vi "Send VmaxVmin Notifier.vi"(8 "error in (no error)":errorcluster, 9 "VmaxVmin Range":string, 10 "Channel":string) -> (0 "error out":errorcluster)   [LabVIEW 2015]
uses:
  DAQ Engine VIs/PXI Globals.vi
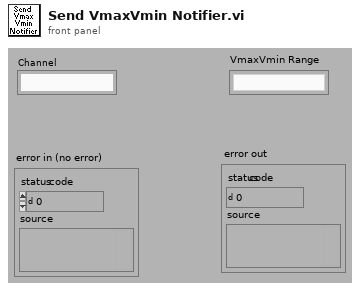
[diagram p1: front panel]
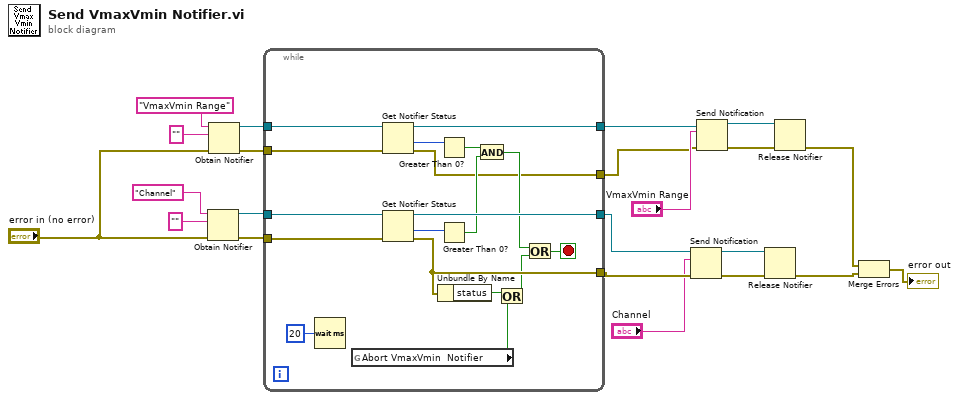
[diagram p0: block diagram]
diagram:
  n1 = Obtain Notifier(name (unnamed)="Channel", notification data type="" ("Channel 2"), error in (no error)="error in (no error)") -> (notifier out=w14:refnum<notifier>, error out=w13:errorcluster)  [unwired: 1 in, 1 out]
  n2 = Obtain Notifier(name (unnamed)="VmaxVmin Range", notification data type="" ("Channel 2"), error in (no error)="error in (no error)") -> (notifier out=w9:refnum<notifier>, error out=w10:errorcluster)  [unwired: 1 in, 1 out]
  n3 = while {
    tunnel: w14 -> [w39]
    tunnel: w13 -> [w38]
    tunnel: [w36] -> w15
    tunnel: [w26] -> w16
    tunnel: w10 -> [w33]
    tunnel: w9 -> [w32]
    tunnel: [w28] -> w5
    tunnel: [w27] -> w4
    stop <- w35 stop-if-true
    n4 = Wait (ms)(milliseconds to wait=20) -> ()  [unwired: 1 out]
    n5 = global read "PXI Globals.vi" "Abort VmaxVmin  Notifier"() -> (w24:bool)
    n6 = Get Notifier Status(notifier=w32, error in (no error)=w33) -> (notifier out=w28:refnum<notifier>, # waiting=w34:i32, error out=w27:errorcluster)  [unwired: 2 out]
    n7 = Get Notifier Status(notifier=w39, error in (no error)=w38) -> (notifier out=w36:refnum<notifier>, # waiting=w37:i32, error out=w26:errorcluster)  [unwired: 2 out]
    n8 = Unbundle By Name(w26) -> ("status"=w25:bool)
    n9 = Greater Than 0?(x=w34) -> (x > 0?=w31:bool)
    n10 = Greater Than 0?(x=w37) -> (x > 0?=w30:bool)
    n11 = And(x=w31, y=w30) -> (x .and. y?=w29:bool)
    n12 = Or(x=w25, y=w24) -> (x .or. y?=w23:bool)
    n13 = Or(x=w29, y=w23) -> (x .or. y?=w35:bool)
  }
  n14 = Send Notification(notification="Channel", notifier=w15, error in (no error)=w16) -> (notifier out=w17:refnum<notifier>, error out=w18:errorcluster)
  n15 = Send Notification(notification="VmaxVmin Range", notifier=w5, error in (no error)=w4) -> (notifier out=w7:refnum<notifier>, error out=w8:errorcluster)
  n16 = Release Notifier(notifier=w17, error in (no error)=w18) -> (error out=w2:errorcluster)  [unwired: 1 in, 2 out]
  n17 = Release Notifier(notifier=w7, error in (no error)=w8) -> (error out=w1:errorcluster)  [unwired: 1 in, 2 out]
  n18 = Merge Errors(w1, w2) -> (→"error out":errorcluster)
